vi "Read Double Direct Dispatch.vi"(8 "error in (no error)":errorcluster, 9 "Timeout (ms)":i32, 11 "CIFTag in":refnum<class "CIFChannels.lvclass">) -> (0 "error out":errorcluster, 1 "timed out?":bool, 2 "Data":dbl, 3 "CIFTag out":refnum<class "CIF_NIChn_Double.lvclass">)   [LabVIEW 2021, in "CIF_NIChn_Double.lvclass"]
uses:
  CIF_NIChn_Double.lvclass
  CIF_NIChn_Double.lvclass/CIF_NIChn_Double.ctl
  CIFChannels/Typedef/Direction.ctl
  CIFChannels/CIFChannels.lvclass
  CIFChannels/Typedef/Channel State.ctl
  NIChn/CIF_NIChn.lvclass
  D:/dev/Packages/Channel_Manager/src/CIF_NIChn/NIChn/CIF_NIChn.lvclass
  d7866fd0-95aa-4020-8d43-a7942dcd60c7.vi
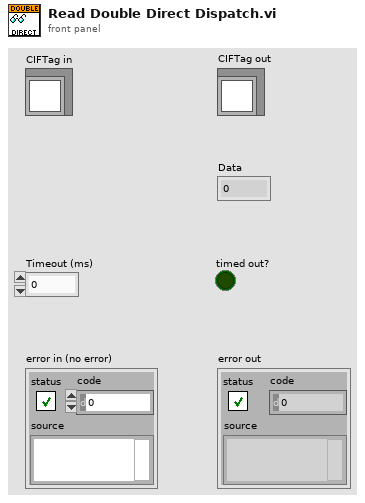
[diagram p1: front panel]
types:
  T1 = typedef "CIFChannels.lvclass/Channel State.ctl" = enum16{"Creating", "Disconnected", "Connecting", "Connected", "Destroyed"}
  T2 = typedef "CIFChannels.lvclass/Direction.ctl" = enum16{"Publisher", "Subscriber"}
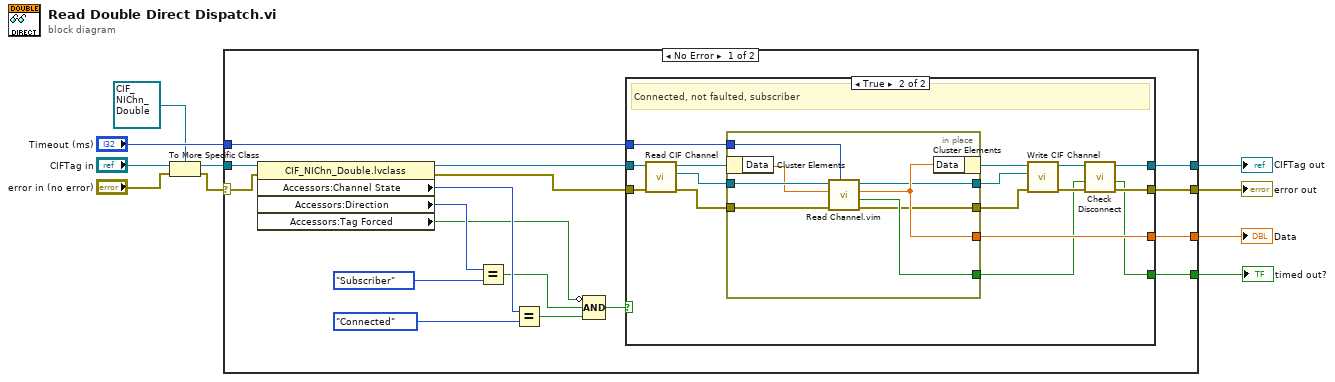
[diagram p0: block diagram]
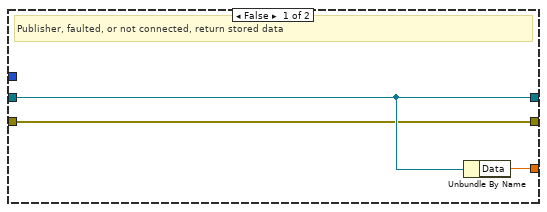
[diagram p2: hidden frame]
diagram:
  n1 = To More Specific Class(target class=refnum<class "CIF_NIChn_Double.lvclass"> refnum ("CIFTag in"), reference="CIFTag in", error in="error in (no error)") -> (specific class reference=w3:refnum<class "CIF_NIChn_Double.lvclass">, error out=w1:errorcluster)
  n2 = case shown="No Error" w1 {
    selector: w1 -> [w24 w56]
    tunnel: [w13 w56] -> w10
    tunnel: [w14 w55] -> w9
    tunnel: w3 -> [w25 w55]
    tunnel: [w27 _] -> w8
    tunnel: [w26 _] -> w7
    tunnel: "Timeout (ms)" -> [w12 _]
    frame No Error {
      n3 = property class="CIF_NIChn_Double.lvclass"(reference=w25, error in=w24) -> (reference out=w23:refnum<class "CIF_NIChn_Double.lvclass">, error out=w22:errorcluster, "Accessors:Channel State"=w19:T1, "Accessors:Direction"=w21:T2, "Accessors:Tag Forced"=w11:bool)
      n4 = Equal?(x=w21, y=Direction."Subscriber") -> (x = y?=w15:bool)
      n5 = Equal?(x=w19, y=Channel_State."Connected") -> (x = y?=w17:bool)
      n6 = Compound Arithmetic op=AND(invert w11, w15, w17) -> (w16:bool)
      n7 = case shown="True" w16 {
        tunnel: [_ w32] -> w27
        tunnel: [w30 w39] -> w26
        tunnel: w22 -> [w28 w45]
        tunnel: w23 -> [w29 w46]
        tunnel: [w29 w44] -> w14
        tunnel: [w28 w43] -> w13
        tunnel: w12 -> [_ w31]
        frame False {
          # "Publisher, faulted, or not connected, return stored data"
          n8 = Unbundle By Name(w29) -> ("Data"=w30:dbl)
        }
        frame True {
          # "Connected, not faulted, subscriber"
          n9 = call "Read CIF Channel.vi"("error in (no error)"=w45, "CIFTag in"=w46) -> ("error out"=w40:errorcluster, "CIF Channel"=w41:refnum<k21>, "CIFTag out"=w42:refnum<class "CIF_NIChn_Double.lvclass">)  [unwired: 7 in]
          n10 = in-place {
            in-place-border: [w51] -> w33
            in-place-border: w41 -> [w54]
            in-place-border: w40 -> [w52]
            in-place-border: [w50] -> w39
            in-place-border: [w49] -> w36
            in-place-border: [w48] -> w37
            in-place-border: w31 -> [w47]
            n11 = in-place-cluster #1(w42) -> ("Data"=w53:dbl)
            n12 = call "Read Channel.vim"("Timeout (ms)"=w47, "error in"=w52, "Data in"=w53, "CIF Channel in"=w54) -> ("error out"=w48:errorcluster, "Timed out?"=w51:bool, "Data out"=w50:dbl, "CIF Channel out"=w49:refnum<k21>)  [unwired: 4 in]
            n13 = in-place-cluster #1("Data"=w50) -> (w38:refnum<class "CIF_NIChn_Double.lvclass">)
          }
          n14 = call "Write CIF Channel.vi"("error in (no error)"=w37, "CIF Channel"=w36, "CIFTag in"=w38) -> ("error out"=w34:errorcluster, "CIFTag out"=w35:refnum<class "CIF_NIChn_Double.lvclass">)  [unwired: 7 in]
          n15 = call "Check Disconnect.vi"("error in (no error)"=w34, "timeout in"=w33, "CIFTag in"=w35) -> ("error out"=w43:errorcluster, "timeout out"=w32:bool, "CIFTag out"=w44:refnum<class "CIF_NIChn_Double.lvclass">)  [unwired: 5 in, 1 out]
        }
      }
    }
    frame Error {
    }
  }
  "error out" <- w10
  "CIFTag out" <- w9
  "timed out?" <- w8
  "Data" <- w7
